vi "Get New Level.vi"(8 "error in (no error)":cluster{"状态":bool, "代码":i32, "源":string} caption="错误输入（无错误）", 11 "冷却器输入":refnum<class "Cooler.lvclass">) -> (0 "error out":cluster{"状态":bool, "代码":i32, "源":string} caption="错误输出", 2 "水位":dbl, 3 "冷却器输出":refnum<class "Cooler.lvclass">)   [LabVIEW 2015, in "Cooler.lvlib" / "Cooler.lvclass"]
doc: "子类不应对该VI进行重写。如子类需要对该VI进行重写，则必须采用“调用父项”节点。"
uses:
  Cooler.lvclass
  Cooler.lvclass/Cooler.ctl
  Cooler Controller/Update Current Temperature Msg/Update Current Temperature Msg.lvclass/Update Current Temperature Msg.ctl
  <vilib>/ActorFramework/Message Enqueuer/Message Enqueuer.lvclass/Message Enqueuer.ctl
  <vilib>/ActorFramework/Message Enqueuer/Enqueue.vi
  <vilib>/ActorFramework/Message Priority Queue/Priority Enqueue.vi
  Cooler Controller/Update Current Temperature Msg/Update Current Temperature Msg.lvclass
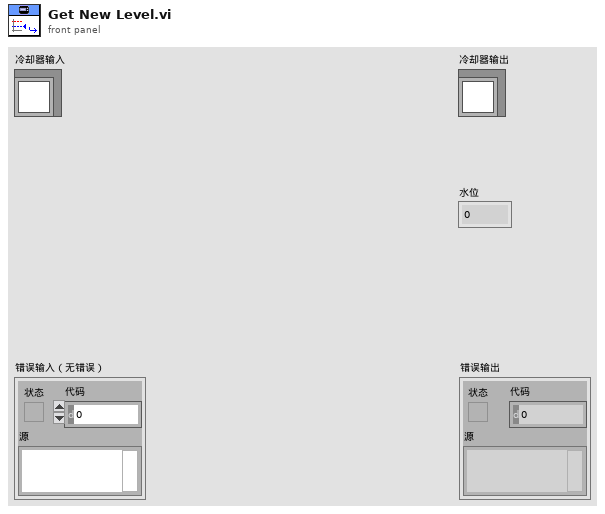
[diagram p1: front panel]
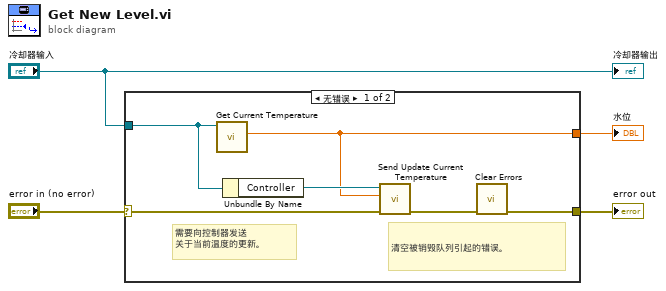
[diagram p0: block diagram]
diagram:
  n1 = case shown="无错误" "error in (no error)" {
    selector: "error in (no error)" -> [w7 w11]
    tunnel: "冷却器输入" -> [w10 _]
    tunnel: [w8 _] -> w3
    tunnel: [w5 w11] -> w2
    frame No Error {
      # "清空被销毁队列引起的错误。"
      # "需要向控制器发送\n关于当前温度的更新。"
      n2 = call-dynamic "Get Current Temperature.vi"("冷却器输入"=w10) -> ("水位"=w8:dbl)  [unwired: 9 in, 1 out]
      n3 = Unbundle By Name(w10) -> ("Controller"=w9:refnum<class "Message Enqueuer.lvclass">)
      n4 = call "Send Update Current Temperature.vi"("error in (no error)"=w7, "当前温度"=w8, "消息待入队列"=w9) -> ("error out"=w6:cluster{"状态":bool, "代码":i32, "源":string})  [unwired: 8 in]
      n5 = call <vilib>:"Clear Errors.vi"("error in (no error)"=w6) -> ("error out"=w5:errorcluster)  [unwired: 5 in, 1 out]
    }
    frame Error {
    }
  }
  "error out" <- w2
  "水位" <- w3
  "冷却器输出" <- "冷却器输入"
